vi "UpdateLEDSettingsFromFile.vi"(9 "name or relative path":string="2016LED", 10 "LED Color Ref":refnum<vi>, 11 "Path Ref":refnum<vi>) -> (3 "dup path":path)   [LabVIEW 2015]
uses:
  <vilib>/Utility/sysdir.llb/System Directory Type.ctl
  <vilib>/Utility/file.llb/Read Delimited Spreadsheet (string).vi
panel:
  out "error out":errorcluster
  in  "error in (no error)":errorcluster
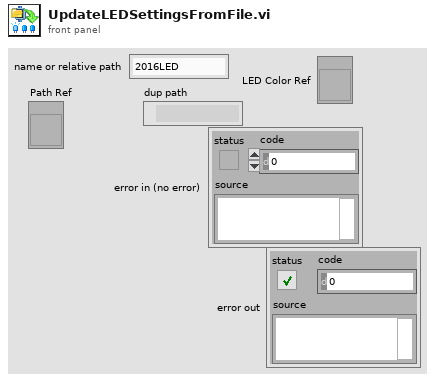
[diagram p1: front panel]
types:
  T1 = cluster{"Hue":cluster{dbl, dbl}, "Sat":cluster{dbl, dbl}, "Val":cluster{dbl, dbl}}
  T2 = typedef "System Directory Type.ctl" = i32
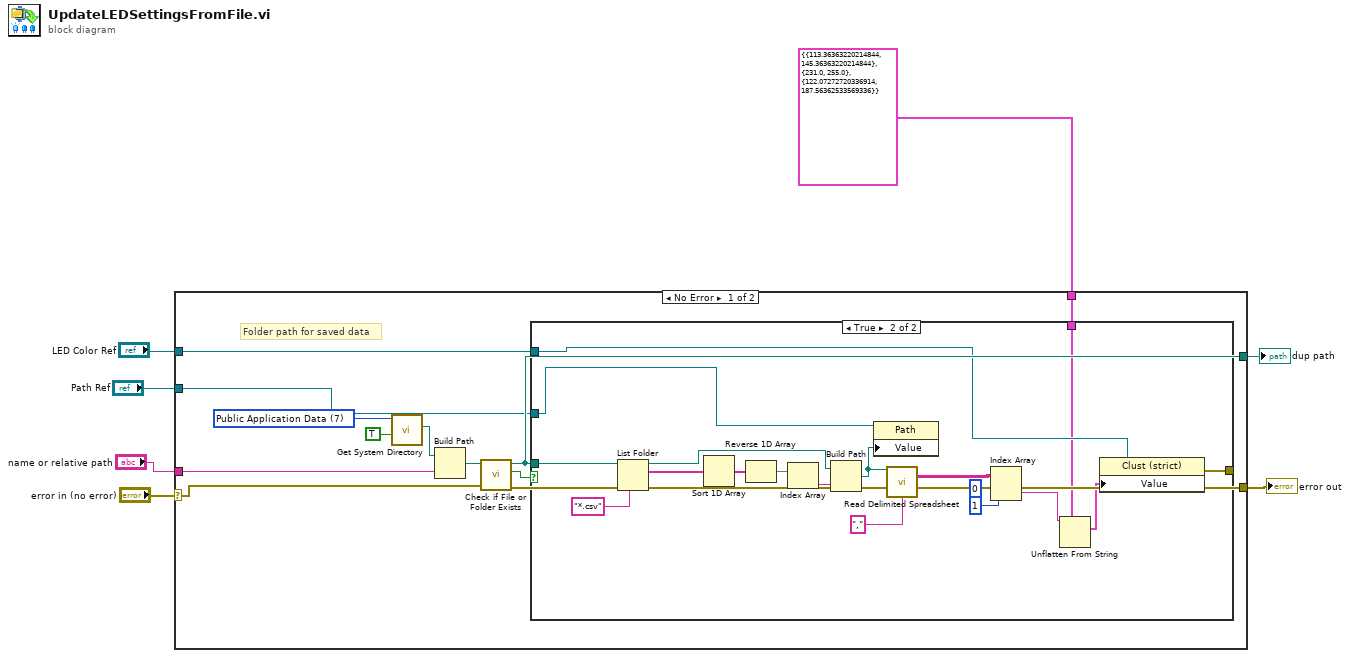
[diagram p0: block diagram]
diagram:
  n1 = case shown="No Error" "error in (no error)" {
    selector: "error in (no error)" -> [w11 w38]
    tunnel: "LED Color Ref" -> [w19 _]
    tunnel: [w18 _] -> w7
    tunnel: "Path Ref" -> [w12 _]
    tunnel: [w10 w38] -> w4
    tunnel: "name or relative path" -> [w9 _]
    tunnel: T1 {"Hue"={113.36363220214844, 145.36363220214844}, "Sat"={231.0, 255.0}, "Val"={122.07272720336914, 187.56362533569336}} ("LED Color") -> [w8 _]
    frame No Error {
      w14 = T2 7 items=["User Home"=0, "User Desktop"=1, "User Documents"=2, "User Application Data"=3, "User Preferences"=4, "User Temporary"=5, "Public Documents"=6, "Public Application Data"=7, "Public Preferences"=8, "Public Cache"=13, "System Core Libraries"=9, "System Installed Libraries"=10, "Application Files"=11, "Boot Volume Root"=12] ("system directory type")
      # "Folder path for saved data"
      n2 = call <vilib>:"Get System Directory.vi"("create directory if not found? (F)"=TRUE, "system directory type"=w14) -> ("system directory"=w15:path)  [unwired: 9 in]
      n3 = Build Path(base path=w15, name or relative path=w9) -> (appended path=w13:path)
      n4 = call <vilib>:"Check if File or Folder Exists.vi"("error in (no error)"=w11, "path"=w13) -> ("error out"=w10:errorcluster, "file or folder exists?"=w17:bool, "dup path"=w18:path)  [unwired: 7 in]
      n5 = case shown="True" w17 {
        tunnel: w18 -> [_ w37]
        tunnel: w19 -> [_ w30]
        tunnel: [_ w29] -> _
        tunnel: w12 -> [_ w28]
        tunnel: w8 -> [_ w21]
        frame False {
        }
        frame True {
          n6 = List Folder(path=w37, pattern="*.csv") -> (path out=w31:path, filenames=w35:string[])  [unwired: 2 in, 2 out]
          n7 = Sort 1D Array(array=w35) -> (sorted array=w34:string[])
          n8 = Reverse 1D Array(array=w34) -> (reversed array=w33:string[])
          n9 = Index Array(array=w33) -> (element=w32:string)  [unwired: 1 in]
          n10 = Build Path(base path=w31, name or relative path=w32) -> (appended path=w27:path)
          n11 = property class="Path"(reference=w28, "Value"=w27) -> ()  [unwired: 1 in, 2 out]
          n12 = call-poly <vilib>:"Read Delimited Spreadsheet.vi"("file path (dialog if empty)"=w27, "delimiter (\\t)"="," ("delimiter (\\t)")) -> ("all rows"=w25:string[][])  [unwired: 8 in, 5 out]
          n13 = Index Array(array=w25, index (row)=0, index (col)=1 ("disabled index (col)")) -> (element=w22:string)
          n14 = Unflatten From String(type=w21, binary string=w22) -> (value=w20:T1)  [unwired: 3 in, 2 out]
          n15 = property class="Clust (strict)"(reference=w30, "Value"=w20) -> (error out=w29:errorcluster)  [unwired: 1 in, 1 out]
        }
      }
    }
    frame Error {
    }
  }
  "dup path" <- w7
  "error out" <- w4
